vi "Kronecker Product.vi"   [LabVIEW 2024, in "NI_AALPro.lvlib"]
doc: "<p>Calculates the Kronecker product of the input matrices <strong>A</strong> and <strong>B</strong>. The data types you wire to the <strong>A</strong> and <strong>B</strong> inputs determine the polymorphic instance to use.</p>"
uses:
  NI_AALPro.lvlib
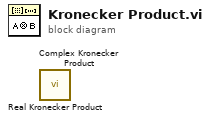
[diagram p0: block diagram]
diagram:
  n1 = call "Real Kronecker Product.vi"() -> ()  [unwired: 10 in, 2 out]
  n2 = call "Complex Kronecker Product.vi"() -> ()  [unwired: 10 in, 2 out]
